vi "uMsg Get CMD.vi"(8 "error in (no error)":errorcluster, 11 "uMsg in":refnum<class "uMsg.lvclass">) -> (0 "error out":errorcluster, 2 "CMD":string, 3 "uMsg out":refnum<class "uMsg.lvclass">)   [LabVIEW 2023, in "uLib.lvlib" / "uMsg.lvclass"]
uses:
  uMsg.lvclass
  uMsg.lvclass/uMsg.ctl
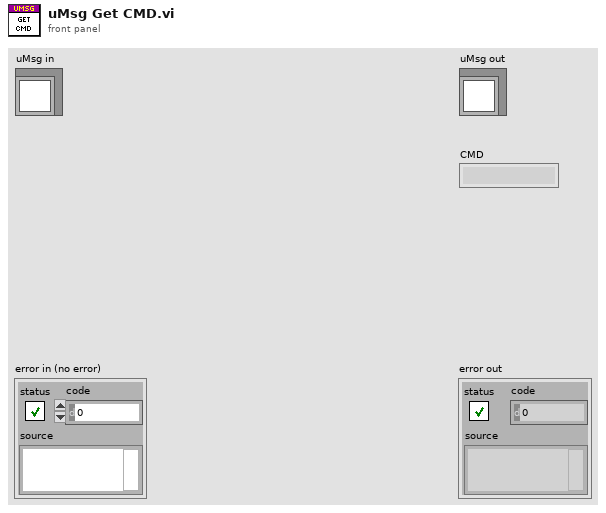
[diagram p1: front panel]
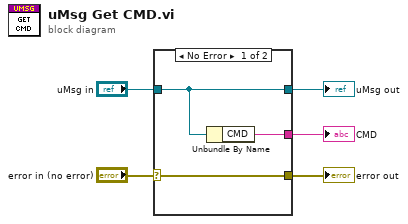
[diagram p0: block diagram]
diagram:
  n1 = case shown="No Error" "error in (no error)" {
    selector: "error in (no error)" -> [w6 w9]
    tunnel: [w8 _] -> w5
    tunnel: "uMsg in" -> [w7 w10]
    tunnel: [w7 w10] -> w3
    tunnel: [w6 w9] -> w1
    frame No Error {
      n2 = Unbundle By Name(w7) -> ("CMD"=w8:string)
    }
    frame Error {
    }
  }
  "error out" <- w1
  "uMsg out" <- w3
  "CMD" <- w5
